vi "Update ILC Rate.vi"(8 "error in (no error)":errorcluster, 11 "Model in":refnum<class "Model.lvclass">) -> (0 "error out":errorcluster, 3 "Model out":refnum<class "Model.lvclass">)   [LabVIEW 2015, in "Model.lvclass"]
uses:
  Model.lvclass
  Model.lvclass/Model.ctl
  <userlib>/Common/ILC/ILC/ILC.lvclass/ILC.ctl
  <userlib>/Common/ILC/ILC/ILC.lvclass
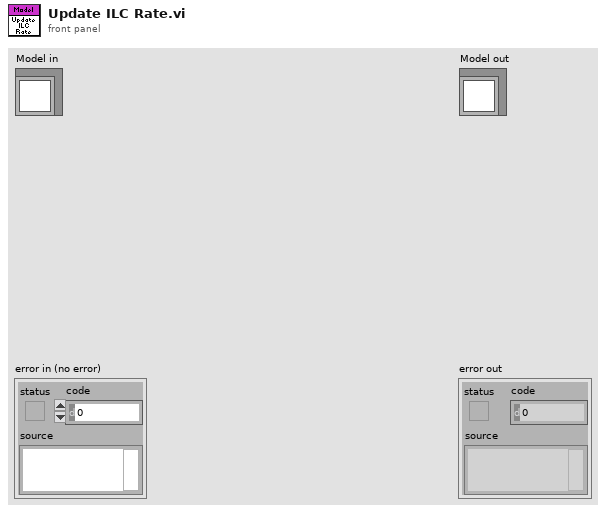
[diagram p1: front panel]
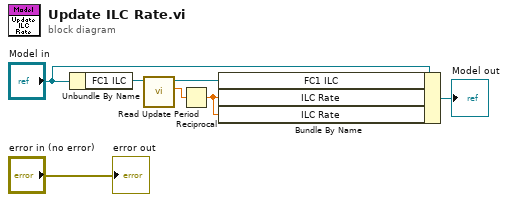
[diagram p0: block diagram]
diagram:
  n1 = Unbundle By Name("Model in") -> ("FC1 ILC"=w6:refnum<class "ILC.lvclass">)
  n2 = call <userlib>:"Read Update Period.vi"("ILC in"=w6) -> ("Update Period"=w5:dbl[unit], "ILC out"=w1:refnum<class "ILC.lvclass">)  [unwired: 9 in]
  n3 = Reciprocal(x=w5) -> (1/x=w2:dbl[unit])
  n4 = Bundle By Name(cluster="Model in", "FC1 ILC"=w1, "ILC Rate"=w2, "ILC Rate"=w2) -> (→"Model out":refnum<class "Model.lvclass">)
  "error out" <- "error in (no error)"
